vi "Global 4.vi"() -> ()   [LabVIEW 2015]
panel:
  out "error out":errorcluster
  in  "error in (no error)":errorcluster
  in  "String":string
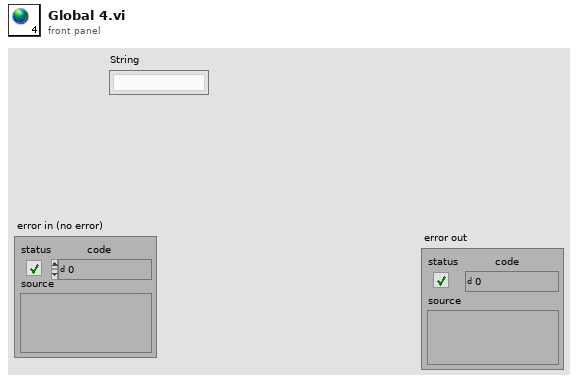
[diagram p1: front panel]
diagram:
